vi "LabvolutionSubmoduleCheck_GitCommit.vi"(8 "error in (no error)":errorcluster, 10 "Message":string, 11 "Working Dir in":path) -> (0 "error out":errorcluster, 2 "Command OK":bool, 3 "Working Dir out":path)   [LabVIEW 2018]
uses:
  callback-system-exec/callback-system-exec/callback-system-exec.lvlib
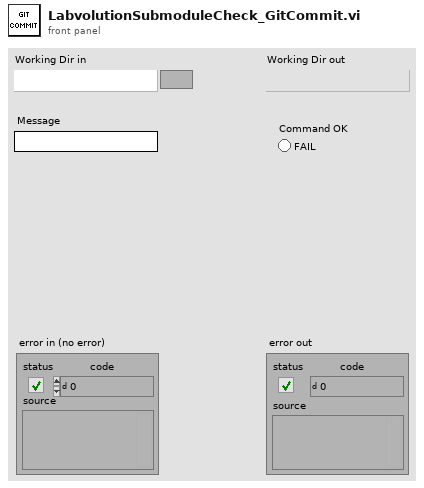
[diagram p1: front panel]
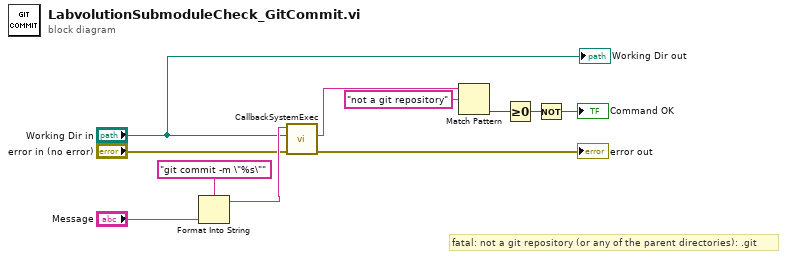
[diagram p0: block diagram]
diagram:
  # "fatal: not a git repository (or any of the parent directories): .git"
  n1 = Format Into String(format string="git commit -m \"%s\"", "Message") -> (resulting string=w3:string)  [unwired: 2 in, 1 out]
  n2 = call "CallbackSystemExec.vi"("error in (no error)"="error in (no error)", "Working directory"="Working Dir in", "Command"=w3) -> ("error out"=→"error out":errorcluster, "Standard Error"=w4:string)  [unwired: 6 in, 1 out]
  n3 = Match Pattern(string=w4, regular expression="not a git repository") -> (offset past match=w10:i32)  [unwired: 1 in, 3 out]
  n4 = Greater Or Equal To 0?(x=w10) -> (x >= 0?=w9:bool)
  n5 = Not(x=w9) -> (.not. x?=→"Command OK":bool)
  "Working Dir out" <- "Working Dir in"
